vi "waveout.vi"() -> ()   [LabVIEW 2011]
uses:
  Windows/System32/winmm.dll
panel:
  out "pwoc":T1
  out "return type":i32
  in  "error in (no error)":errorcluster
  out "error out":errorcluster
  out "dwSupport 2":u32
  in  "dwSupport":u32
  in  "cbwoc":u32=48
  in  "WaveOutCaps":T1
  # "typedef struct tagWAVEINCAPSA {\n    WORD    wMid;                    /* manufacturer ID */\n    WORD    wPid;                    /* product ID */\n    MMVERSION vDriverVersion;        /* version of the driver */\n    CHAR    szPname[MAXPNAMELEN];    /* product name (NULL terminated string) */\n    DWORD   dwFormats;               /* formats supported */\n    WORD    wChannels;               /* number of channels supported */\n    WORD    wReserved1;              /* structure packing */\n} WAVEINCAPSA, *PWAVEINCAPSA, *NPWAVEINCAPSA, *LPWAVEINCAPSA;"
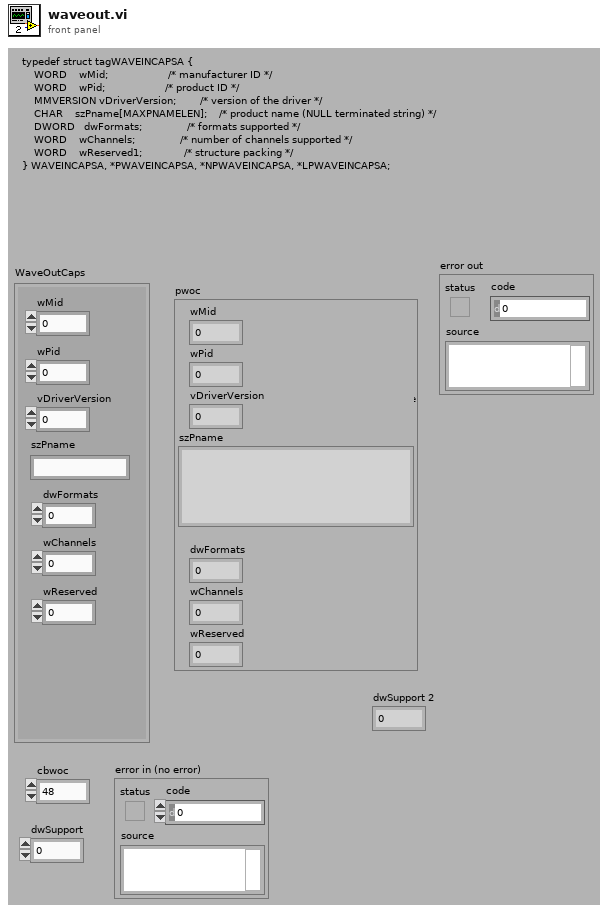
[diagram p1: front panel]
types:
  T1 = cluster{"wMid":u16, "wPid":u16, "vDriverVersion":u32, "szPname":string, "dwFormats":u32, "wChannels":u16, "wReserved":u16}
  T2 = cluster{"U*8 Array[0]":u8, "U*8 Array[1]":u8, "U*8 Array[2]":u8, "U*8 Array[3]":u8, "U*8 Array[4]":u8, "U*8 Array[5]":u8, "U*8 Array[6]":u8, "U*8 Array[7]":u8, "U*8 Array[8]":u8, "U*8 Array[9]":u8, "U*8 Array[10]":u8, "U*8 Array[11]":u8, "U*8 Array[12]":u8, "U*8 Array[13]":u8, "U*8 Array[14]":u8, "U*8 Array[15]":u8, "U*8 Array[16]":u8, "U*8 Array[17]":u8, "U*8 Array[18]":u8, "U*8 Array[19]":u8, "U*8 Array[20]":u8, "U*8 Array[21]":u8, "U*8 Array[22]":u8, "U*8 Array[23]":u8, "U*8 Array[24]":u8, "U*8 Array[25]":u8, "U*8 Array[26]":u8, "U*8 Array[27]":u8, "U*8 Array[28]":u8, "U*8 Array[29]":u8, "U*8 Array[30]":u8, "U*8 Array[31]":u8}
  T3 = cluster{"wMid":u16, "wPid":u16, "vDriverVersion":u32, "U*8 Array":cluster{"U*8 Array[0]":u8, "U*8 Array[1]":u8, "U*8 Array[2]":u8, "U*8 Array[3]":u8, "U*8 Array[4]":u8, "U*8 Array[5]":u8, "U*8 Array[6]":u8, "U*8 Array[7]":u8, "U*8 Array[8]":u8, "U*8 Array[9]":u8, "U*8 Array[10]":u8, "U*8 Array[11]":u8, "U*8 Array[12]":u8, "U*8 Array[13]":u8, "U*8 Array[14]":u8, "U*8 Array[15]":u8, "U*8 Array[16]":u8, "U*8 Array[17]":u8, "U*8 Array[18]":u8, "U*8 Array[19]":u8, "U*8 Array[20]":u8, "U*8 Array[21]":u8, "U*8 Array[22]":u8, "U*8 Array[23]":u8, "U*8 Array[24]":u8, "U*8 Array[25]":u8, "U*8 Array[26]":u8, "U*8 Array[27]":u8, "U*8 Array[28]":u8, "U*8 Array[29]":u8, "U*8 Array[30]":u8, "U*8 Array[31]":u8}, "dwFormats":u32, "wChannels":u16, "wReserved":u16}
  T4 = cluster{"wMid":u16, "wPid":u16, "vDriverVersion":u32, string, "dwFormats":u32, "wChannels":u16, "wReserved":u16}
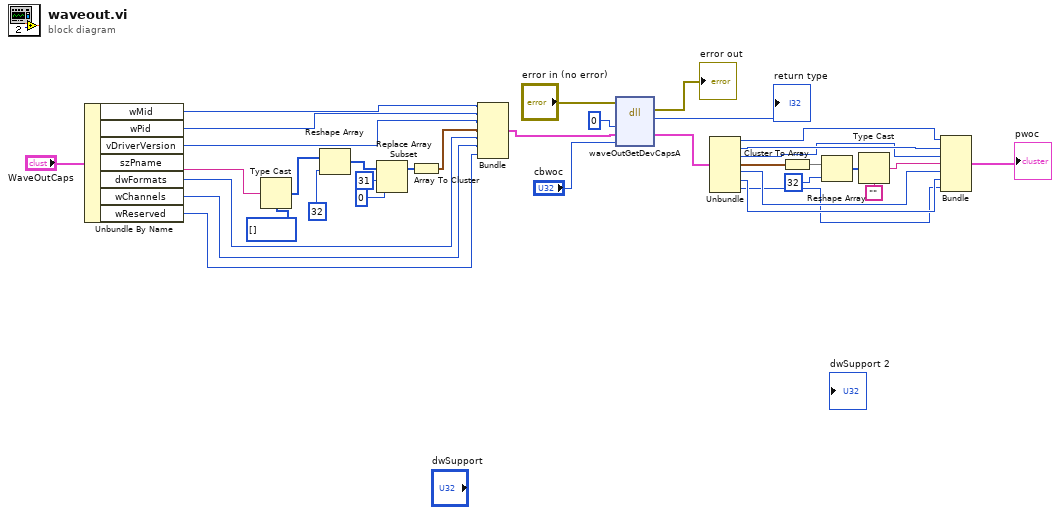
[diagram p0: block diagram]
diagram:
  n1 = Unbundle By Name("WaveOutCaps") -> ("wMid"=w8:u16, "wPid"=w7:u16, "vDriverVersion"=w6:u32, "szPname"=w26:string, "dwFormats"=w4:u32, "wChannels"=w3:u16, "wReserved"=w2:u16)
  n2 = Type Cast(type=u8[] [] ("U*8 Array"), x=w26) -> (*(type *) &x=w27:u8[])
  n3 = Reshape Array(w27, 32 ("dimension size")) -> (w29:u8[])
  n4 = Replace Array Subset(array=w29, new element=u8 0 ("new element/subarray"), index=31) -> (w9:u8[])
  n5 = Array To Cluster(array=w9) -> (cluster=w5:T2)
  n6 = Bundle("wMid"=w8, "wPid"=w7, "vDriverVersion"=w6, "U*8 Array"=w5, "dwFormats"=w4, "wChannels"=w3, "wReserved"=w2) -> (w1:T3)  [unwired: 1 in]
  n7 = dll-call lib="C:/Windows/System32/winmm.dll" fn="waveOutGetDevCapsA"(error in="error in (no error)", "uDeviceID"=u32 0, "pwoc"=w1, "cbwoc"="cbwoc") -> (error out=→"error out":errorcluster, "return type"=→"return type":i32, "pwoc"=w22:T3)  [unwired: 4 in, 1 out]
  n8 = Unbundle(w22) -> ("wMid"=w17:u16, "wPid"=w16:u16, "vDriverVersion"=w15:u32, "U*8 Array"=w21:T2, "dwFormats"=w14:u32, "wChannels"=w13:u16, "wReserved"=w12:u16)
  n9 = Cluster To Array(cluster=w21) -> (array=w23:u8[])
  n10 = Reshape Array(w23, 32 ("x")) -> (w20:u8[])
  n11 = Type Cast(type="", x=w20) -> (*(type *) &x=w18:string)
  n12 = Bundle("wMid"=w17, "wPid"=w16, "vDriverVersion"=w15, w18, "dwFormats"=w14, "wChannels"=w13, "wReserved"=w12) -> (→"pwoc":T4)  [unwired: 1 out]
